vi "Ignore-error-custom.vi"(8 "error in (no error)":errorcluster, 10 "Error to ignore":T1=enum."State not implemented") -> (0 "error out":errorcluster)   [LabVIEW 2013, in "Error-handling.lvlib" / "Errors.lvclass"]
uses:
  Errors.lvclass
  Custom-errors.ctl
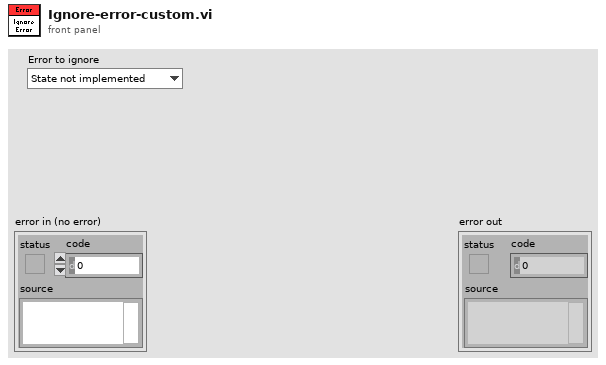
[diagram p1: front panel]
types:
  T1 = typedef "Error-handling.lvlib/Errors.lvclass/Custom-errors.ctl" = enum16{"No error", "State not implemented", "Initialization failed", "Language not implemented", "Error not implemented"}
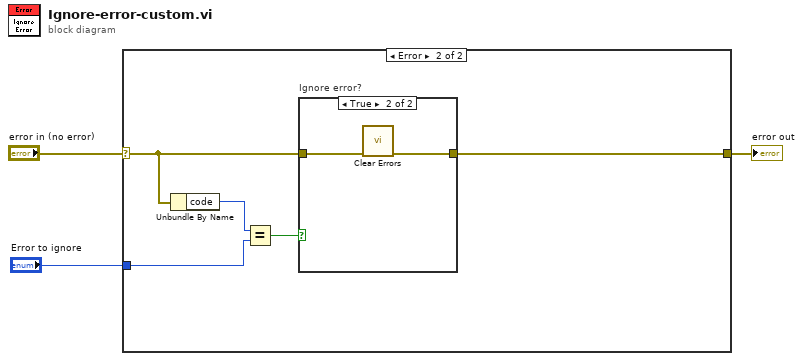
[diagram p0: block diagram]
diagram:
  n1 = case shown="Error" "error in (no error)" {
    selector: "error in (no error)" -> [w4 w6]
    tunnel: [w4 w5] -> w2
    tunnel: "Error to ignore" -> [_ w8]
    frame No Error {
    }
    frame Error {
      n2 = Unbundle By Name(w6) -> ("code"=w9:i32)
      n3 = Equal?(x=w9, y=w8) -> (x = y?=w7:bool)
      n4 = case "Ignore error?" shown="True" w7 {
        tunnel: w6 -> [w10 w12]
        tunnel: [w10 w11] -> w5
        frame False {
        }
        frame True {
          n5 = call <vilib>:"Clear Errors.vi"("error in (no error)"=w12) -> ("error out"=w11:errorcluster)  [unwired: 6 in]
        }
      }
    }
  }
  "error out" <- w2
